vi "Find Classes.vi"(8 "error in (no error)":errorcluster, 11 "Component Loader in":refnum<class "Component Loader.lvclass">) -> (0 "error out":errorcluster, 2 "class paths":path[](array[path]), 3 "Component Loader out":refnum<class "Component Loader.lvclass">)   [LabVIEW 2017, in "Data Sharing Framework Core.lvlib" / "Data Sharing Framework Engine.lvlib" / "Component Loader.lvclass"]
uses:
  Component Loader.lvclass
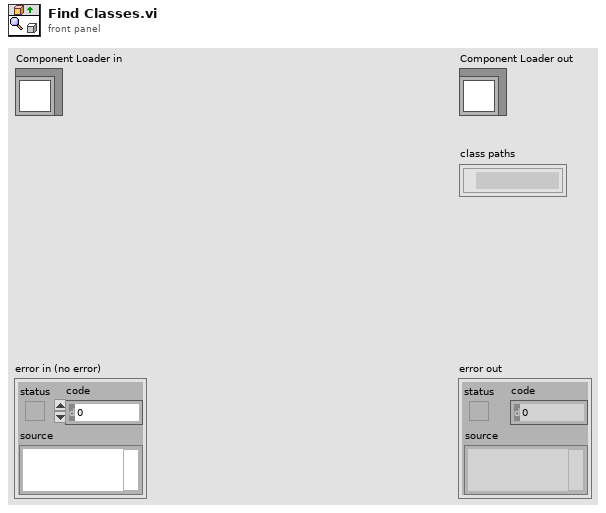
[diagram p1: front panel]
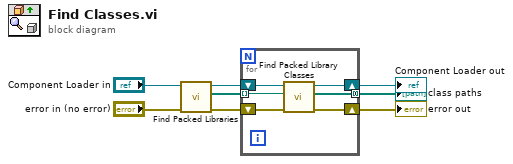
[diagram p0: block diagram]
diagram:
  n1 = call "Find Packed Libraries.vi"("error in (no error)"="error in (no error)", "Component Loader in"="Component Loader in") -> ("error out"=w6:errorcluster, "packed library paths"=w1:path[], "Component Loader out"=w3:refnum<class "Component Loader.lvclass">)  [unwired: 7 in]
  n2 = for {
    tunnel: [w12] -> w4 mode=concatenating
    tunnel: w1 -> [w9] mode=indexing
    shift-right: [w13] -> w5
    shift-left: w6 -> [w14]
    shift-right: [w10] -> w2
    shift-left: w3 -> [w11]
    n3 = call "Find Packed Library Classes.vi"("error in (no error)"=w14, "packed library path"=w9, "Component Loader in"=w11) -> ("error out"=w13:errorcluster, "class paths"=w12:path[], "Component Loader out"=w10:refnum<class "Component Loader.lvclass">)  [unwired: 6 in]
  }
  "error out" <- w5
  "Component Loader out" <- w2
  "class paths" <- w4
